vi "TCP-Get Local Address.vi"() -> (8 "net address":u32, 10 "address":string)   [LabVIEW 2020]
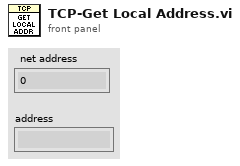
[diagram p1: front panel]
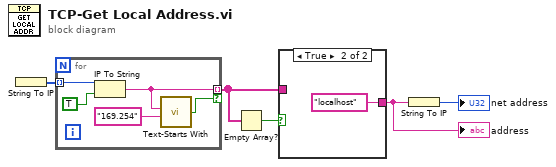
[diagram p0: block diagram]
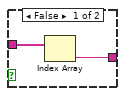
[diagram p2: hidden frame]
diagram:
  n1 = String To IP() -> (0:w1:u32[])  [unwired: 1 in]
  n2 = for {
    tunnel: w1 -> [w9] mode=indexing
    tunnel: [w8] -> w3 mode=indexing if=w7
    n3 = IP To String(1:TRUE ("dot notation? (F)"), 2:w9) -> (0:w8:string)
    n4 = call "Text-Starts With.vi"("Starts with"="169.254", "String"=w8) -> ("result"=w7:bool)  [unwired: 4 in]
  }
  n5 = Empty Array?(array=w3) -> (empty?=w4:bool)
  n6 = case shown="True" w4 {
    tunnel: w3 -> [w12 _]
    tunnel: [w11 "localhost"] -> w5
    frame False {
      n7 = Index Array(array=w12) -> (element=w11:string)  [unwired: 1 in]
    }
    frame True {
    }
  }
  "address" <- w5
  n8 = String To IP(1:w5) -> (0:→"net address":u32)
